vi "Part 1.vi"(11 "Input":string) -> (3 "Output":i64)   [LabVIEW 2021]
uses:
  <userlib>/_OpenG.lib/string/string.llb/Convert EOLs (String)__ogtk.vi
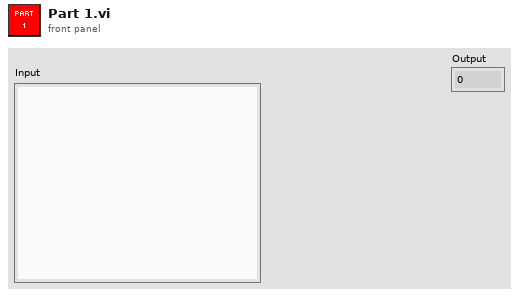
[diagram p1: front panel]
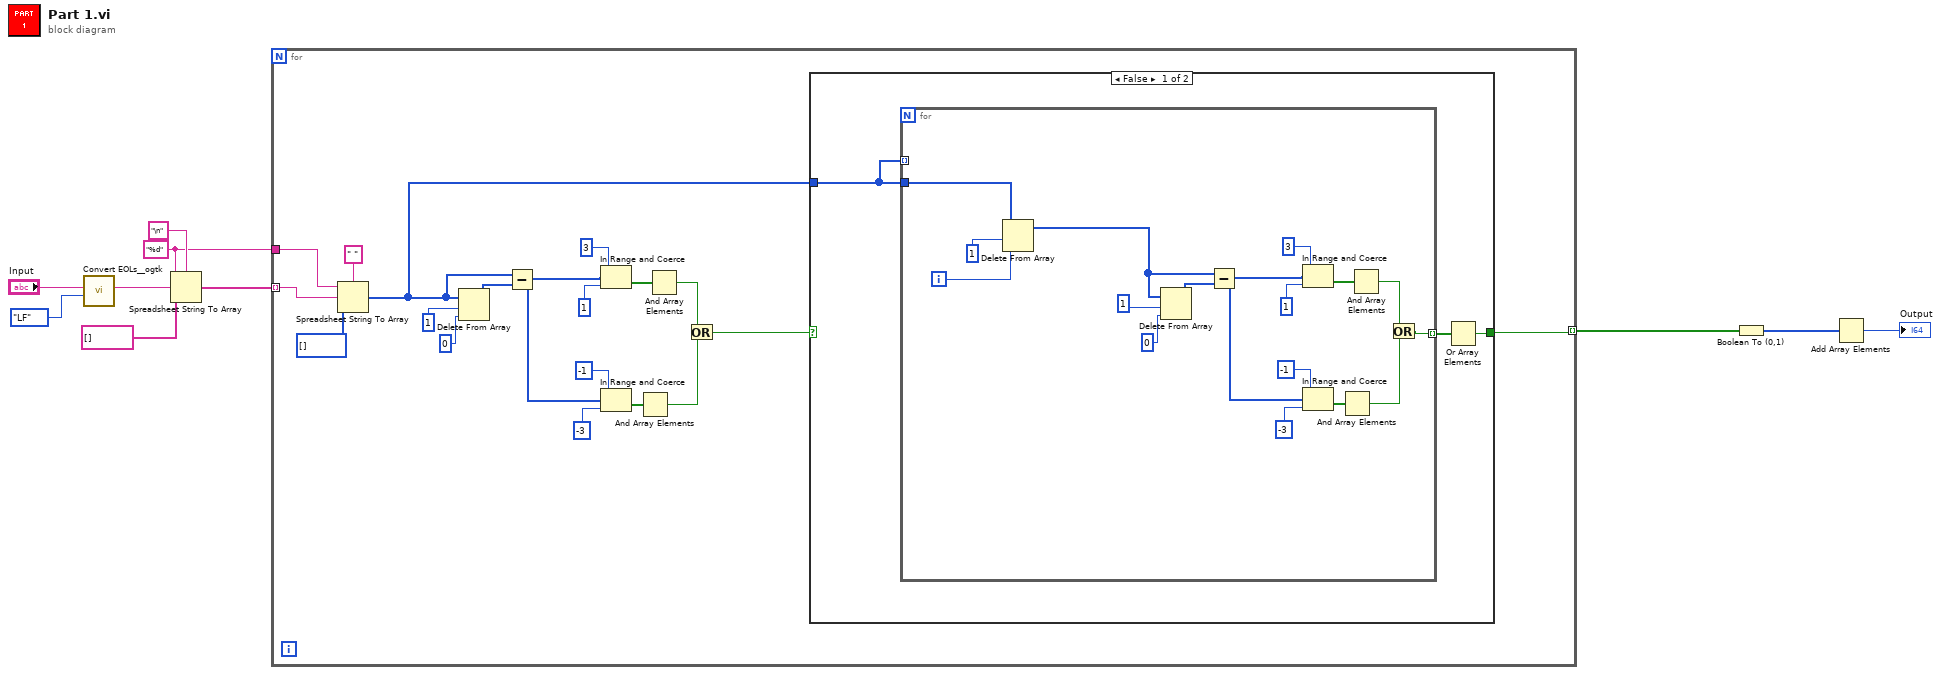
[diagram p0: block diagram]
diagram:
  w3 = "%d"
  n1 = call-poly <userlib>:"Convert EOLs__ogtk.vi"("Convert to:"=enum16{"CR", "LF", "CRLF"}."LF", "String in"="Input") -> ("String out"=w8:string)  [unwired: 9 in]
  n2 = Spreadsheet String To Array(delimiter (Tab)="\n", format string=w3, spreadsheet string=w8, array type (2D Dbl)=string[] []) -> (array=w6:string[])
  n3 = for {
    tunnel: w6 -> [w21] mode=indexing
    tunnel: [w12] -> w5 mode=indexing
    tunnel: w3 -> [w20]
    n4 = Spreadsheet String To Array(delimiter (Tab)=" ", format string=w20, spreadsheet string=w21, array type (2D Dbl)=i64[] []) -> (array=w11:i64[])
    n5 = Delete From Array(array=w11, length=1 ("index"), index=0) -> (array with subset deleted=w25:i64[])  [unwired: 1 out]
    n6 = Subtract(x=w11, y=w25) -> (x-y=w17:i64[])
    n7 = In Range and Coerce(upper limit=3 ("index"), x=w17, lower limit=1 ("index")) -> (In Range?=w22:bool[])  [unwired: 1 out]
    n8 = In Range and Coerce(upper limit=-1 ("index"), x=w17, lower limit=-3 ("index")) -> (In Range?=w16:bool[])  [unwired: 1 out]
    n9 = And Array Elements(Boolean array=w16) -> (logical AND=w14:bool)
    n10 = And Array Elements(Boolean array=w22) -> (logical AND=w15:bool)
    n11 = Or(x=w15, y=w14) -> (x .or. y?=w13:bool)
    n12 = case shown="False" w13 {
      selector: w13 -> [_ w50]
      tunnel: [w30 w50] -> w12
      tunnel: w11 -> [w32 _]
      frame False {
        n13 = for {
          tunnel: w32 -> [w36]
          tunnel: w32 -> [_] mode=indexing
          tunnel: [w38] -> w31 mode=indexing
          i -> [w35]
          n14 = Delete From Array(array=w36, length=1 ("index"), index=w35) -> (array with subset deleted=w34:i64[])  [unwired: 1 out]
          n15 = Delete From Array(array=w34, length=1 ("index"), index=0) -> (array with subset deleted=w48:i64[])  [unwired: 1 out]
          n16 = Subtract(x=w34, y=w48) -> (x-y=w42:i64[])
          n17 = In Range and Coerce(upper limit=3 ("index"), x=w42, lower limit=1 ("index")) -> (In Range?=w45:bool[])  [unwired: 1 out]
          n18 = In Range and Coerce(upper limit=-1 ("index"), x=w42, lower limit=-3 ("index")) -> (In Range?=w41:bool[])  [unwired: 1 out]
          n19 = And Array Elements(Boolean array=w41) -> (logical AND=w39:bool)
          n20 = And Array Elements(Boolean array=w45) -> (logical AND=w40:bool)
          n21 = Or(x=w40, y=w39) -> (x .or. y?=w38:bool)
        }
        n22 = Or Array Elements(Boolean array=w31) -> (logical OR=w30:bool)
      }
      frame True {
      }
    }
  }
  n23 = Boolean To (0,1)(Boolean=w5) -> (0, 1=w2:i16[])
  n24 = Add Array Elements(numeric array=w2) -> (sum=→"Output":i16)
